vi "SVI_TD_Parser.vi"(0 "read buffer":string, 1 "Time Step (ms)":i32, 3 "In":T1) -> (5 "Current Values":T2, 8 "Out":T1)   [LabVIEW 2014]
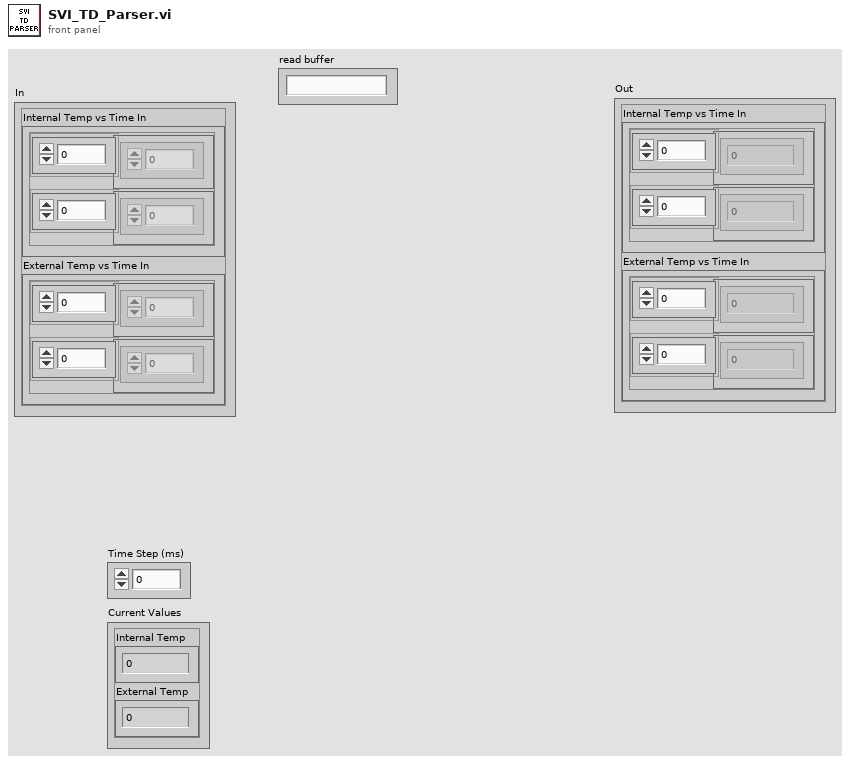
[diagram p1: front panel]
types:
  T1 = cluster{"Internal Temp vs Time In":cluster{"Array":dbl[], "Array":dbl[]}, "External Temp vs Time In":cluster{"Array":dbl[], "Array":dbl[]}}
  T2 = cluster{"Internal Temp":dbl, "External Temp":dbl}
  T3 = cluster{cluster{dbl[], dbl[]}, cluster{dbl[], dbl[]}}
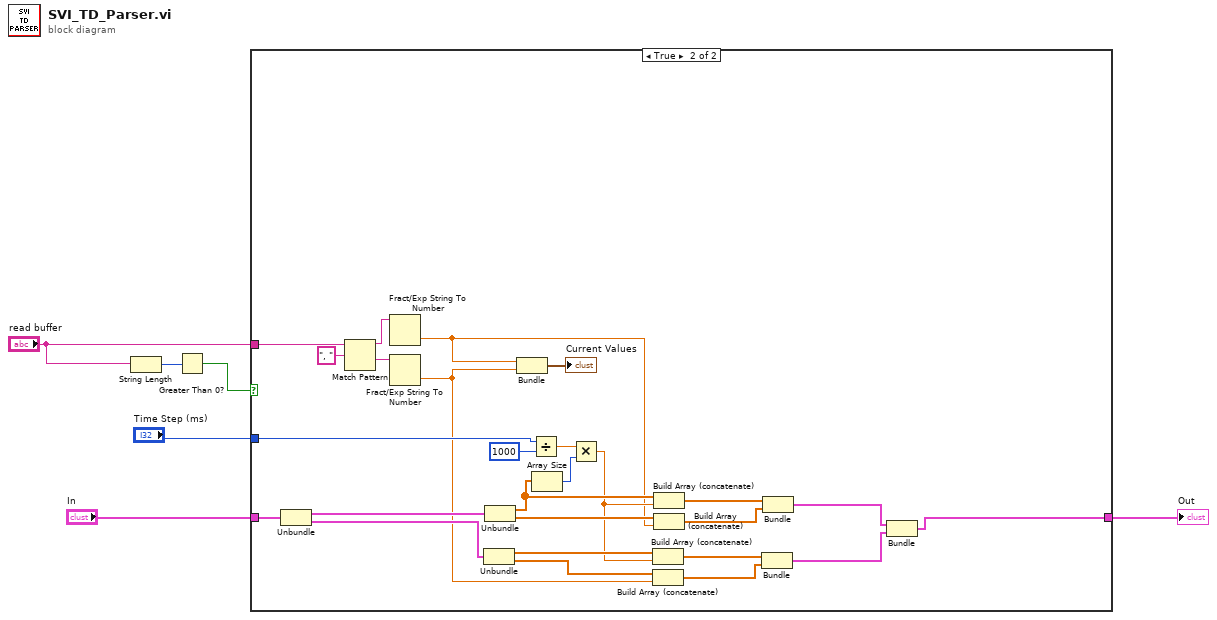
[diagram p0: block diagram]
diagram:
  n1 = String Length(string="read buffer") -> (length=w6:i32)
  n2 = Greater Than 0?(x=w6) -> (x > 0?=w5:bool)
  n3 = case shown="True" w5 {
    tunnel: "read buffer" -> [_ w29]
    tunnel: "Time Step (ms)" -> [_ w20]
    tunnel: "In" -> [w7 w33]
    tunnel: [w7 w13] -> w1
    frame False {
    }
    frame True {
      n4 = Unbundle(w33) -> ("Internal Temp vs Time In"=w21:cluster{"Array":dbl[], "Array":dbl[]}, "External Temp vs Time In"=w12:cluster{"Array":dbl[], "Array":dbl[]})
      n5 = Match Pattern(string=w29, regular expression=", ") -> (before substring=w31:string, after substring=w30:string)  [unwired: 1 in, 2 out]
      n6 = Fract/Exp String To Number(string=w31) -> (number=w9:dbl)  [unwired: 3 in, 1 out]
      n7 = Fract/Exp String To Number(string=w30) -> (number=w10:dbl)  [unwired: 3 in, 1 out]
      n8 = Unbundle(w12) -> ("Array"=w17:dbl[], "Array"=w15:dbl[])
      n9 = Unbundle(w21) -> ("Array"=w24:dbl[], "Array"=w26:dbl[])
      n10 = Bundle(w9, w10) -> (→"Current Values":cluster{dbl, dbl})  [unwired: 1 in]
      n11 = Divide(x=w20, y=1000) -> (x/y=w27:dbl)
      n12 = Array Size(array=w24) -> (size(s)=w23:i32)
      n13 = Multiply(x=w27, y=w23) -> (x*y=w11:dbl)
      n14 = Build Array (concatenate)(w17, w11) -> (w18:dbl[])
      n15 = Build Array (concatenate)(w15, w10) -> (w16:dbl[])
      n16 = Build Array (concatenate)(w24, w11) -> (w22:dbl[])
      n17 = Build Array (concatenate)(w26, w9) -> (w25:dbl[])
      n18 = Bundle(w18, w16) -> (w14:cluster{dbl[], dbl[]})  [unwired: 1 in]
      n19 = Bundle(w22, w25) -> (w19:cluster{dbl[], dbl[]})  [unwired: 1 in]
      n20 = Bundle(w19, w14) -> (w13:T3)  [unwired: 1 in]
    }
  }
  "Out" <- w1
